vi "h5_2D_I32_stacking.vi"(5 "max_repeats":i32=-1, 6 "Attributes":variant, 7 "TYPE":string="IMG", 8 "error in (no error)":errorcluster, 9 "2D I32":i32[][](array[numeric]), 10 "SQUID":string="1", 11 "H5":path[](array[path])) -> (0 "error out":errorcluster, 2 "Exists":bool)   [LabVIEW 2013]
uses:
  <vilib>/addons/h5labview2/file/H5Fmode.ctl
  <vilib>/addons/h5labview2/base/lib_path.vi
  <vilib>/addons/h5labview2/base/H5Equery.vi
  <vilib>/addons/h5labview2/dataset/H5Dwrite.llb/H5Dwrite.xnode
  <vilib>/addons/h5labview2/base/hid_t.ctl
  <vilib>/addons/h5labview2/file/H5F.lvlib
  <vilib>/addons/h5labview2/group/H5G.lvlib
  <vilib>/addons/h5labview2/dataset/H5D.lvlib
  <vilib>/addons/h5labview2/attrib/H5A.lvlib
  <vilib>/addons/h5labview2/space/H5S.lvlib
panel:
  out "error out 2":errorcluster
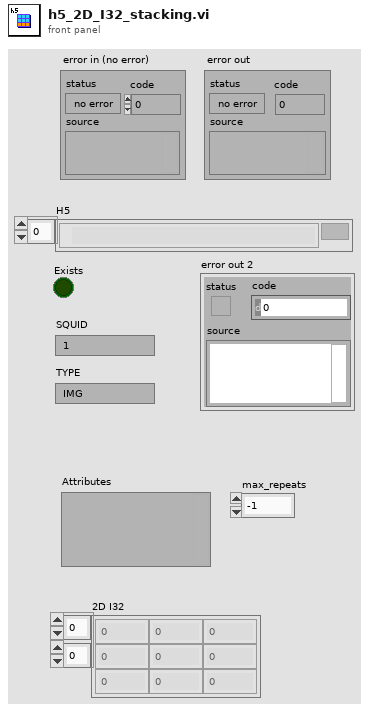
[diagram p1: front panel]
types:
  T1 = typedef "Semaphore RefNum" = refnum<k1>
  T2 = typedef "H5F.lvlib/H5Fmode.ctl" = enum16{"read-only", "read-write", "overwrite", "create new", "open or create"}
  T3 = typedef "hid_t.ctl" = i32
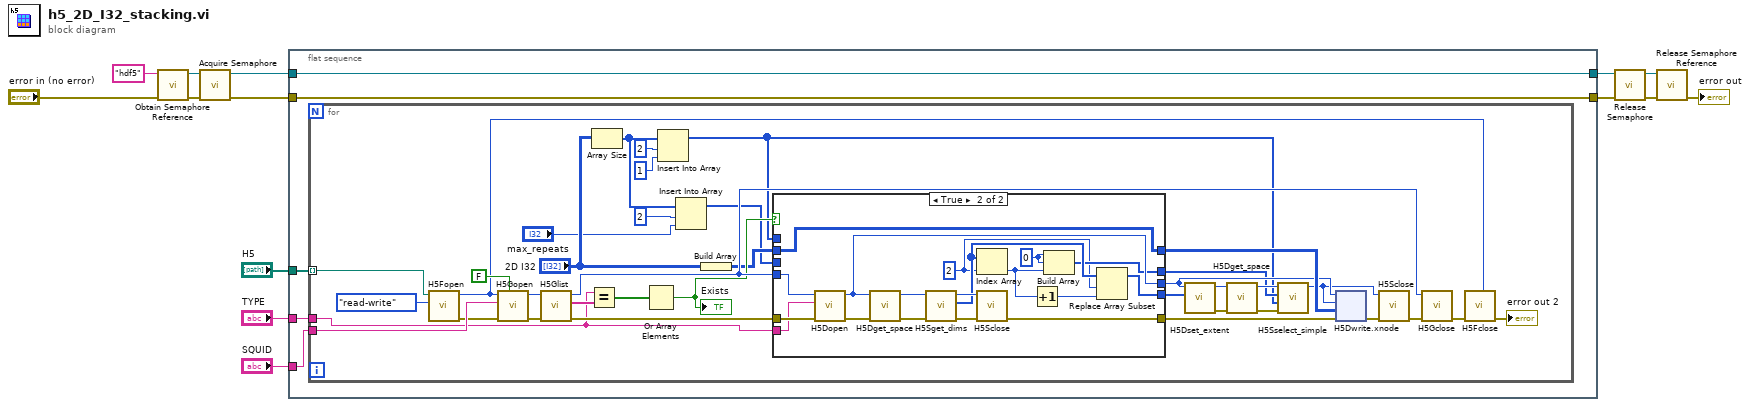
[diagram p0: block diagram]
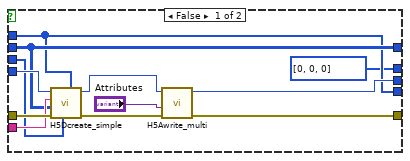
[diagram p2: hidden frame]
diagram:
  n1 = call <vilib>:"Obtain Semaphore Reference.vi"("error in (no error)"="error in (no error)", "name (unnamed)"="hdf5") -> ("error out"=w13:errorcluster, "semaphore"=w14:T1)  [unwired: 3 in, 1 out]
  n2 = call <vilib>:"Acquire Semaphore.vi"("error in (no error)"=w13, "semaphore"=w14) -> ("error out"=w7:errorcluster, "semaphore out"=w6:T1)  [unwired: 3 in, 1 out]
  n3 = flat-sequence {
    tunnel: [w19] -> w8
    tunnel: w7 -> [w19]
    tunnel: w6 -> [w18]
    tunnel: [w18] -> w5
    tunnel: "H5" -> [w17]
    tunnel: "SQUID" -> [w16]
    tunnel: "TYPE" -> [w15]
    frame #0 {
      n4 = for {
        tunnel: w17 -> [w48] mode=indexing
        tunnel: w16 -> [w49]
        tunnel: w15 -> [w40]
        n5 = call <vilib>:"H5Fopen.vi"("mode (read-only)"=H5Fmode."read-write", "path"=w48) -> ("error out"=w47:errorcluster, "ref out"=w46:T3)  [unwired: 8 in]
        n6 = call <vilib>:"H5Gopen.vi"("create? (F)"=FALSE, "error in (no error)"=w47, "name"=w49, "ref in"=w46) -> ("error out"=w44:errorcluster, "group out"=w45:T3)  [unwired: 6 in]
        n7 = call <vilib>:"H5Glist.vi"("error in (no error)"=w44, "ref in"=w45) -> ("error out"=w43:errorcluster, "names"=w41:string[], "ref out"=w42:T3)  [unwired: 6 in, 1 out]
        n8 = Equal?(x=w40, y=w41) -> (x = y?=w39:bool[])
        n9 = Array Size(array="2D I32") -> (size(s)=w32:i32[])
        n10 = Or Array Elements(Boolean array=w39) -> (logical OR=w38:bool)
        "Exists" <- w38
        n11 = Insert Into Array(array=w32, index=2, new element=1 ("new element/subarray")) -> (w21:i32[])
        n12 = Insert Into Array(array=w32, index=2, new element="max_repeats") -> (w29:i32[])
        n13 = Build Array("2D I32") -> (w34:i32[][][])
        n14 = case shown="True" w38 {
          tunnel: w43 -> [w86 w103]
          tunnel: w34 -> [w83 w104]
          tunnel: w42 -> [w85 w101]
          tunnel: w40 -> [w84 w102]
          tunnel: [w77 w96] -> w33
          tunnel: w21 -> [w76 _]
          tunnel: [w83 w104] -> w54
          tunnel: [w78 w94] -> w24
          tunnel: w29 -> [w79 _]
          tunnel: [w76 w91] -> w23
          tunnel: [u64[] [0, 0, 0] ("start") w88] -> w22
          frame False {
            n15 = call <vilib>:"H5Dcreate_simple.vi"("chunk size"=w76, "initial size"=w79, "error in (no error)"=w86, "type in"=w83, "name"=w84, "ref in"=w85) -> ("error out"=w81:errorcluster, "dset out"=w80:T3)  [unwired: 4 in]
            n16 = call <vilib>:"H5Awrite_multi.vi"("error in (no error)"=w81, "variant in"="Attributes", "ref in"=w80) -> ("error out"=w77:errorcluster, "ref out"=w78:T3)  [unwired: 7 in]
          }
          frame True {
            w89 = u64 0 ("element")
            w87 = 2 ("index")
            n17 = call <vilib>:"H5Dopen.vi"("error in (no error)"=w103, "name"=w102, "loc in"=w101) -> ("error out"=w95:errorcluster, "dset out"=w94:T3)  [unwired: 7 in]
            n18 = call <vilib>:"H5Dget_space.vi"("error in (no error)"=w95, "ref in"=w94) -> ("error out"=w100:errorcluster, "space out"=w99:T3)  [unwired: 8 in]
            n19 = call <vilib>:"H5Sget_dims.vi"("error in (no error)"=w100, "space in"=w99) -> ("error out"=w98:errorcluster, "dims"=w92:u32[], "space out"=w97:T3)  [unwired: 6 in, 1 out]
            n20 = Index Array(array=w92, index=w87) -> (element=w90:u32)
            n21 = call <vilib>:"H5Sclose.vi"("error in (no error)"=w98, "space in"=w97) -> ("error out"=w96:errorcluster)  [unwired: 9 in]
            n22 = Increment(x=w90) -> (x+1=w93:u32)
            n23 = Build Array(w89, w89, w90) -> (w88:u64[])
            n24 = Replace Array Subset(array=w92, new element=w93, index=w87) -> (w91:u32[])
          }
        }
        n25 = call <vilib>:"H5Dset_extent.vi"("new size"=w23, "dset in"=w24) -> ("error out"=w28:errorcluster, "dset out"=w27:T3)  [unwired: 8 in]
        n26 = call <vilib>:"H5Dget_space.vi"("error in (no error)"=w28, "ref in"=w27) -> ("error out"=w26:errorcluster, "space out"=w25:T3)  [unwired: 8 in]
        n27 = call <vilib>:"H5Sselect_simple.vi"("error in (no error)"=w26, "count"=w21, "start"=w22, "space in"=w25) -> ("space out"=w20:T3)  [unwired: 6 in, 1 out]
        n28 = xnode "H5Dwrite.xnode"("error in (no error)"=w33, "data"=w54, "file space"=w20, "ref in"=w24) -> ("error out"=w55:errorcluster)  [unwired: 3 in, 2 out]
        n29 = call <vilib>:"H5Sclose.vi"("error in (no error)"=w55, "space in"=w20) -> ("error out"=w52:errorcluster)  [unwired: 9 in]
        n30 = call <vilib>:"H5Gclose.vi"("error in (no error)"=w52, "group in"=w42) -> ("error out"=w50:errorcluster)  [unwired: 9 in]
        n31 = call <vilib>:"H5Fclose.vi"("error in (no error)"=w50, "ref"=w46) -> ("error out"=→"error out 2":errorcluster)  [unwired: 9 in]
      }
    }
  }
  n32 = call <vilib>:"Release Semaphore.vi"("error in (no error)"=w8, "semaphore"=w5) -> ("error out"=w9:errorcluster, "semaphore out"=w10:T1)  [unwired: 4 in]
  n33 = call <vilib>:"Release Semaphore Reference.vi"("error in (no error)"=w9, "semaphore"=w10) -> ("error out"=→"error out":errorcluster)  [unwired: 8 in, 1 out]
